vi "BrowerComponent_Create.vi"(6 "SymbolIndex":i32, 8 "error in (no error)":errorcluster, 9 "ComponentName":string, 10 "ComponentID":string, 11 "reference in":refnum<class "BrowerComponent.lvclass">) -> (0 "error out":errorcluster, 3 "reference out":refnum<class "BrowerComponent.lvclass">)   [LabVIEW 2015, in "BrowerComponent.lvclass"]
uses:
  BrowerComponent.lvclass
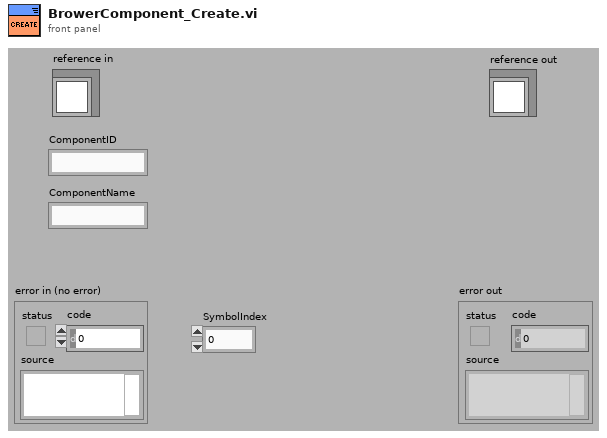
[diagram p1: front panel]
types:
  T1 = typedef "BrowerComponent.lvclass/ObjectAttributes.ctl" = cluster{"ComponentID":string, "SymbolIndex":i32, "ComponentName":string, "PartsOfComponent_dict":variant}
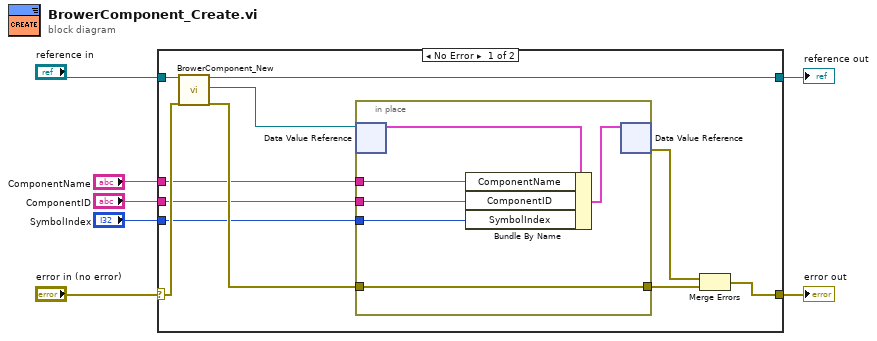
[diagram p0: block diagram]
diagram:
  n1 = case shown="No Error" "error in (no error)" {
    selector: "error in (no error)" -> [w17 w26]
    tunnel: [w14 w26] -> w6
    tunnel: "reference in" -> [w18 w25]
    tunnel: [w16 w25] -> w4
    tunnel: "ComponentName" -> [w10 _]
    tunnel: "ComponentID" -> [w9 _]
    tunnel: "SymbolIndex" -> [w8 _]
    frame No Error {
      n2 = call "BrowerComponent_New.vi"("reference in"=w18, "error in (no error)"=w17) -> ("reference out"=w16:refnum<class "BrowerComponent.lvclass">, "DVRRefOut"=w13:refnum<data-value>, "error out"=w12:errorcluster)  [unwired: 14 in, 1 out]
      n3 = in-place {
        in-place-border: w12 -> [w22]
        in-place-border: [w22] -> w11
        in-place-border: w10 -> [w21]
        in-place-border: w9 -> [w20]
        in-place-border: w8 -> [w19]
        n4 = in-place-dvr #1(w13) -> (w23:T1)  [unwired: 1 out]
        n5 = Bundle By Name(cluster=w23, "ComponentName"=w21, "ComponentID"=w20, "SymbolIndex"=w19) -> (w24:T1)
        n6 = in-place-dvr #1(w24) -> (w15:errorcluster)  [unwired: 1 out]
      }
      n7 = Merge Errors(w15, w11) -> (w14:errorcluster)
    }
    frame Error {
    }
  }
  "error out" <- w6
  "reference out" <- w4
